vi "Publish Status.vi"(6 "Data Type":T1(ring)=enum."string", 8 "error in (no error)":errorcluster, 9 "Value":variant, 10 "Parameter":string, 11 "System Name":string) -> (0 "error out":errorcluster)   [LabVIEW 2024]
doc: "Publishes system status with a shared variable."
uses:
  <vilib>/lvdsc/NI_DSC.lvlib
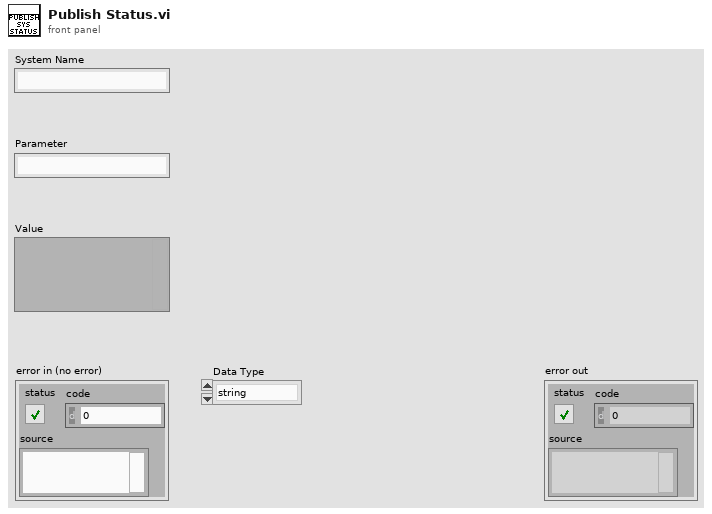
[diagram p1: front panel]
types:
  T1 = enum32{"u32BitField", "bool", "double", "string", "int8", "uint8", "int16", "uint16", "int32", "uint32", "int64", "uint64", "single", "double waveform", "int16 waveform", "array of boolean", "array of int8", "array of uint8", "array of int16", "array of uint16", "array of int32", "array of uint32", "array of int64", "array of uint64", "array of single", "array of double", "array of double waveform", "array of int16 waveform", "array of string", "variant", "timestamp", "fixed point", "custom"}
  T2 = cluster{"enable? (F)":bool, "data type (deprecated)":enum32{"U32 Bit Field", "Boolean", "Double", "String"}, "initial value":variant}
  T3 = cluster{"Read Access":enum8{"Allowed", "Required", "None"}, "Write Access":enum8{"Allowed", "Required", "None"}}
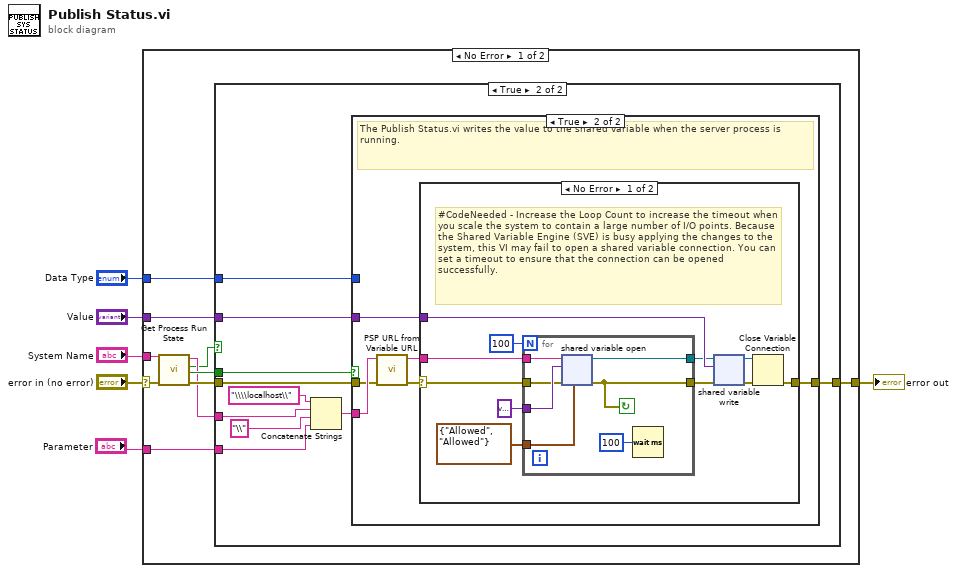
[diagram p0: block diagram]
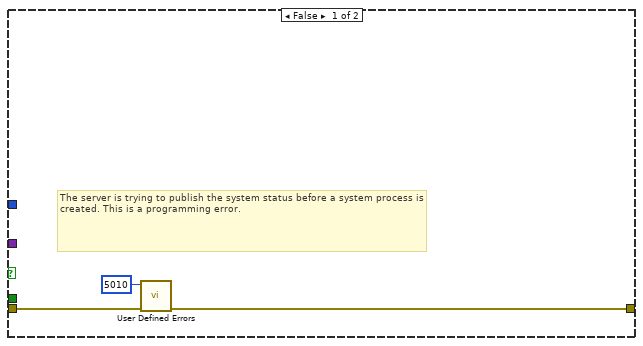
[diagram p2: hidden frame]
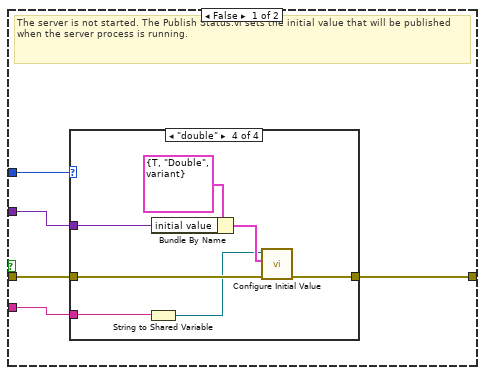
[diagram p3: hidden frame]
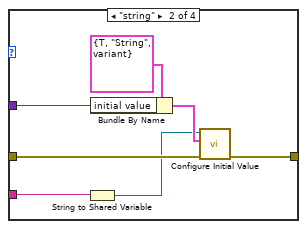
[diagram p5: hidden frame]
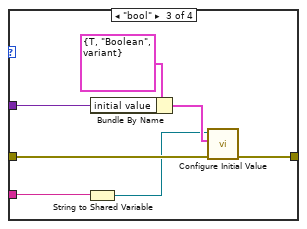
[diagram p6: hidden frame]
diagram:
  n1 = case shown="No Error" "error in (no error)" {
    selector: "error in (no error)" -> [w12 w82]
    tunnel: [w16 w82] -> w5
    tunnel: "System Name" -> [w10 _]
    tunnel: "Parameter" -> [w9 _]
    tunnel: "Value" -> [w8 _]
    tunnel: "Data Type" -> [w7 _]
    frame No Error {
      n2 = call <vilib>:"Get Process Run State.vi"("error in (no error)"=w12, "process name"=w10) -> ("error out"=w15:errorcluster, "running?"=w14:bool, "exists?"=w11:bool, "process name out"=w13:string)  [unwired: 6 in]
      n3 = case shown="True" w11 {
        tunnel: [w18 w29] -> w16
        tunnel: w15 -> [w19 w28]
        tunnel: w14 -> [_ w27]
        tunnel: w13 -> [_ w24]
        tunnel: w9 -> [_ w22]
        tunnel: w8 -> [_ w21]
        tunnel: w7 -> [_ w20]
        frame False {
          # "The server is trying to publish the system status before a system process is created. This is a programming error."
          n4 = call "User Defined Errors.vi"("error in (no error)"=w19, "Error Code (0)"=5010 ("error code (0)")) -> ("error out"=w18:errorcluster)  [unwired: 9 in]
        }
        frame True {
          n5 = Concatenate Strings("\\\\localhost\\" ("string"), w24, "\\" ("string"), w22) -> (w23:string)
          n6 = case shown="True" w27 {
            tunnel: [w34 w62] -> w29
            tunnel: w28 -> [w33 w60]
            tunnel: w23 -> [w31 w61]
            tunnel: w21 -> [w32 w58]
            tunnel: w20 -> [w30 _]
            frame False {
              # "The server is not started. The Publish Status.vi sets the initial value that will be published when the server process is running."
              n7 = case shown="\"double\"" w30 {
                tunnel: [w35 w42 w49 w56] -> w34
                tunnel: w33 -> [w35 w41 w48 w55]
                tunnel: w32 -> [_ w39 w46 w53]
                tunnel: w31 -> [_ w37 w44 w51]
                frame Default {
                }
                frame "string" {
                  n8 = String to Shared Variable(0:w37) -> (2:w36:refnum<k21>)  [unwired: 1 out]
                  n9 = Bundle By Name(cluster=T2 {"enable? (F)"=TRUE, "data type (deprecated)"=enum."String", "initial value"=variant} ("initial value settings"), "initial value"=w39) -> (w38:T2)
                  n10 = call <vilib>:"Configure Initial Value.vi"("error in (no error)"=w41, "initial value settings"=w38, "variable reference in"=w36) -> ("error out"=w42:errorcluster)  [unwired: 7 in, 1 out]
                }
                frame "bool" {
                  n11 = String to Shared Variable(0:w44) -> (2:w43:refnum<k21>)  [unwired: 1 out]
                  n12 = Bundle By Name(cluster=T2 {"enable? (F)"=TRUE, "data type (deprecated)"=enum."Boolean", "initial value"=variant} ("initial value settings"), "initial value"=w46) -> (w45:T2)
                  n13 = call <vilib>:"Configure Initial Value.vi"("error in (no error)"=w48, "initial value settings"=w45, "variable reference in"=w43) -> ("error out"=w49:errorcluster)  [unwired: 7 in, 1 out]
                }
                frame "double" {
                  n14 = String to Shared Variable(0:w51) -> (2:w50:refnum<k21>)  [unwired: 1 out]
                  n15 = Bundle By Name(cluster=T2 {"enable? (F)"=TRUE, "data type (deprecated)"=enum."Double", "initial value"=variant} ("initial value settings"), "initial value"=w53) -> (w52:T2)
                  n16 = call <vilib>:"Configure Initial Value.vi"("error in (no error)"=w55, "initial value settings"=w52, "variable reference in"=w50) -> ("error out"=w56:errorcluster)  [unwired: 7 in, 1 out]
                }
              }
            }
            frame True {
              # "The Publish Status.vi writes the value to the shared variable when the server process is running."
              n17 = call "PSP URL from Variable URL.vi"("error in (no error)"=w60, "Shared Variable URL"=w61) -> ("error out"=w57:errorcluster, "PSP URL"=w59:string)  [unwired: 8 in]
              n18 = case shown="No Error" w57 {
                selector: w57 -> [w63 w81]
                tunnel: [w71 w81] -> w62
                tunnel: w59 -> [w69 _]
                tunnel: w58 -> [w68 _]
                frame No Error {
                  # "#CodeNeeded - Increase the Loop Count to increase the timeout when you scale the system to contain a large number of I/O points. Because the Shared Variable Engine (SVE) is busy applying the changes to the system, this VI may fail to open a shared variable connection. You can set a timeout to ensure that the connection can be opened successfully."
                  n19 = for {
                    N: 100 -> [_]
                    tunnel: T3 {"Read Access"=enum."Allowed", "Write Access"=enum."Allowed"} ("access") -> [w80]
                    tunnel: w69 -> [w79]
                    tunnel: w63 -> [w75]
                    tunnel: variant ("Value") -> [w78]
                    tunnel: [w74] -> w66
                    tunnel: [w77] -> w65
                    stop <- w74 continue-if-true
                    n20 = shared-variable-open(w79, w75, w78, w80) -> (w77:refnum<k21>, w74:errorcluster)
                    n21 = Wait (ms)(milliseconds to wait=u32 100) -> ()  [unwired: 1 out]
                  }
                  n22 = shared-variable-write(w65, w66, w68) -> (w73:refnum<k21>, w72:errorcluster)
                  n23 = Close Variable Connection(8:w72, 11:w73) -> (0:w71:errorcluster)
                }
                frame Error {
                }
              }
            }
          }
        }
      }
    }
    frame Error {
    }
  }
  "error out" <- w5
